vi "publish status.vi"(8 "error in (no error)":errorcluster, 11 "Channel in":refnum<class "Channel.lvclass">) -> (0 "error out":errorcluster, 3 "Channel out":refnum<class "Channel.lvclass">)   [LabVIEW 2018, in "Channel.lvclass"]
uses:
  Channel.lvclass
  Channel.lvclass/Channel.ctl
  State Machine/CCS_State Machine.lvclass/CCS_State Machine.ctl
  State Machine/CCS_State Machine.lvclass
  Simulated_CCD_Camera/Simulated Camera.lvclass
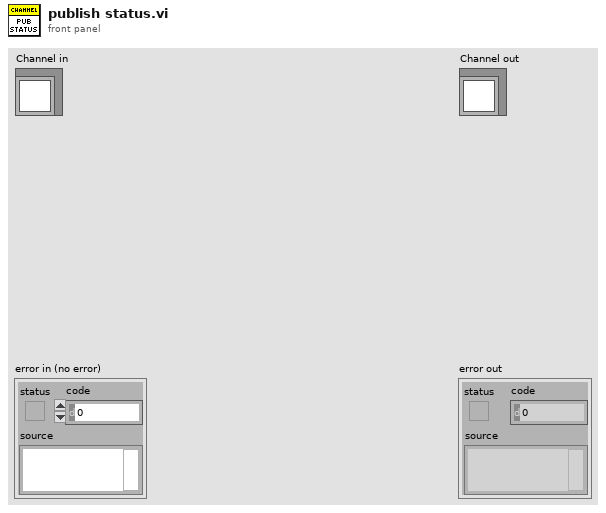
[diagram p1: front panel]
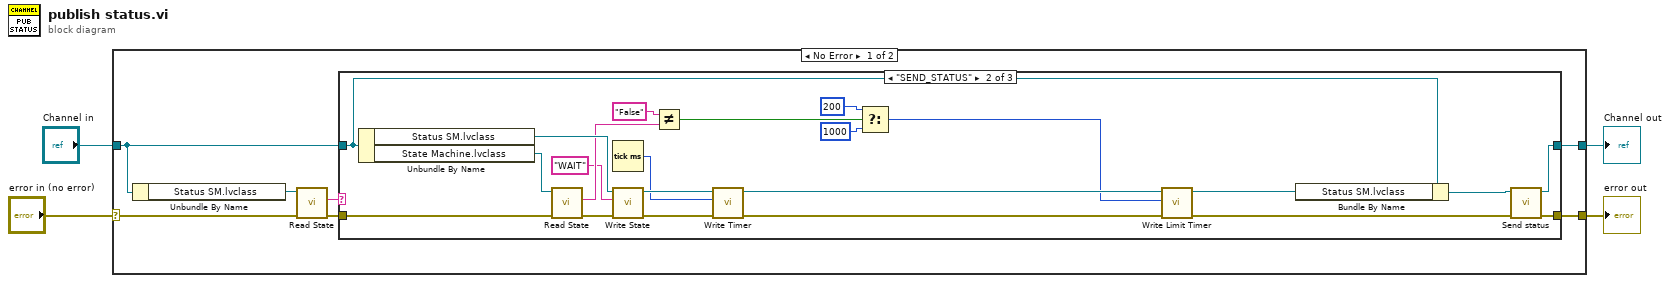
[diagram p0: block diagram]
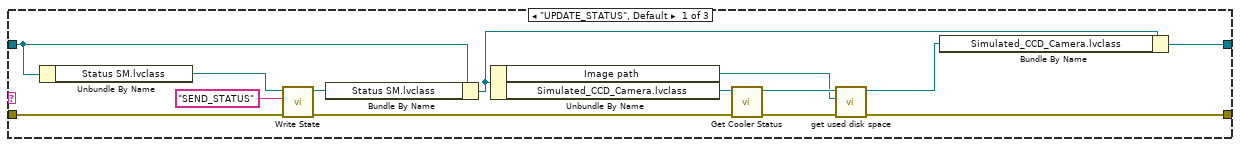
[diagram p2: hidden frame]
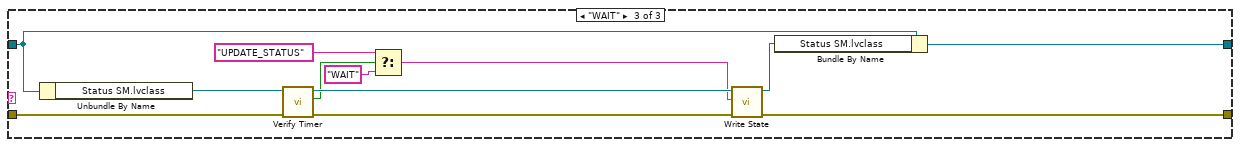
[diagram p3: hidden frame]
diagram:
  n1 = case shown="No Error" "error in (no error)" {
    selector: "error in (no error)" -> [w10 w61]
    tunnel: [w5 w61] -> w3
    tunnel: [w7 w60] -> w1
    tunnel: "Channel in" -> [w6 w60]
    frame No Error {
      n2 = Unbundle By Name(w6) -> ("Status SM.lvclass"=w11:refnum<class "CCS_State Machine.lvclass">)
      n3 = call-dynamic "Read State.vi"("error in (no error)"=w10, "State Machine in"=w11) -> ("error out"=w8:errorcluster, "State"=w9:string)  [unwired: 7 in, 1 out]
      n4 = case shown="\"SEND_STATUS\"" w9 {
        tunnel: w6 -> [w20 w31 w58]
        tunnel: w8 -> [w21 w32 w59]
        tunnel: [w13 w27 w52] -> w5
        tunnel: [w19 w26 w56] -> w7
        frame "UPDATE_STATUS", Default {
          n5 = Unbundle By Name(w20) -> ("Status SM.lvclass"=w23:refnum<class "CCS_State Machine.lvclass">)
          n6 = call-dynamic "Write State.vi"("error in (no error)"=w21, "State"="SEND_STATUS", "State Machine in"=w23) -> ("error out"=w17:errorcluster, "State Machine out"=w24:refnum<class "CCS_State Machine.lvclass">)  [unwired: 7 in]
          n7 = Bundle By Name(cluster=w20, "Status SM.lvclass"=w24) -> (w25:refnum<class "Channel.lvclass">)
          n8 = Unbundle By Name(w25) -> ("Image path"=w12:path, "Simulated_CCD_Camera.lvclass"=w18:refnum<class "Simulated Camera.lvclass">)
          n9 = call-dynamic "Get Cooler Status.vi"("error in (no error)"=w17, "CCDCamera in"=w18) -> ("error out"=w16:errorcluster, "CCDCamera out"=w15:refnum<class "Simulated Camera.lvclass">)  [unwired: 8 in]
          n10 = call "get used disk space.vi"("error in (no error)"=w16, "image path"=w12, "Simulated Camera in"=w15) -> ("error out"=w13:errorcluster, "Simulated Camera out"=w14:refnum<class "Simulated Camera.lvclass">)  [unwired: 7 in]
          n11 = Bundle By Name(cluster=w25, "Simulated_CCD_Camera.lvclass"=w14) -> (w19:refnum<class "Channel.lvclass">)
        }
        frame "SEND_STATUS" {
          n12 = Unbundle By Name(w31) -> ("Status SM.lvclass"=w40:refnum<class "CCS_State Machine.lvclass">, "State Machine.lvclass"=w41:refnum<class "CCS_State Machine.lvclass">)
          n13 = call-dynamic "Read State.vi"("error in (no error)"=w32, "State Machine in"=w41) -> ("error out"=w39:errorcluster, "State"=w38:string)  [unwired: 7 in, 1 out]
          n14 = Tick Count (ms)() -> (millisecond timer value=w45:u32)
          n15 = call-dynamic "Write State.vi"("error in (no error)"=w39, "State"="WAIT", "State Machine in"=w40) -> ("error out"=w46:errorcluster, "State Machine out"=w47:refnum<class "CCS_State Machine.lvclass">)  [unwired: 7 in]
          n16 = Not Equal?(x="False" ("State"), y=w38) -> (x != y?=w30:bool)
          n17 = call "Write Timer.vi"("error in (no error)"=w46, "Timer"=w45, "State Machine in"=w47) -> ("error out"=w42:errorcluster, "State Machine out"=w44:refnum<class "CCS_State Machine.lvclass">)  [unwired: 7 in]
          n18 = Select(t=200, s=w30, f=1000) -> (s? t:f=w37:i32)
          n19 = call "Write Limit Timer.vi"("error in (no error)"=w42, "Limit Timer"=w37, "State Machine in"=w44) -> ("error out"=w28:errorcluster, "State Machine out"=w43:refnum<class "CCS_State Machine.lvclass">)  [unwired: 7 in]
          n20 = Bundle By Name(cluster=w31, "Status SM.lvclass"=w43) -> (w29:refnum<class "Channel.lvclass">)
          n21 = call "Send status.vi"("error in (no error)"=w28, "Channel in"=w29) -> ("error out"=w27:errorcluster, "Channel out"=w26:refnum<class "Channel.lvclass">)  [unwired: 8 in]
        }
        frame "WAIT" {
          n22 = Unbundle By Name(w58) -> ("Status SM.lvclass"=w57:refnum<class "CCS_State Machine.lvclass">)
          n23 = call "Verify Timer.vi"("error in (no error)"=w59, "State Machine in"=w57) -> ("error out"=w55:errorcluster, "time out"=w48:bool, "State Machine out"=w54:refnum<class "CCS_State Machine.lvclass">)  [unwired: 7 in]
          n24 = Select(t="UPDATE_STATUS", s=w48, f="WAIT") -> (s? t:f=w51:string)
          n25 = call-dynamic "Write State.vi"("error in (no error)"=w55, "State"=w51, "State Machine in"=w54) -> ("error out"=w52:errorcluster, "State Machine out"=w53:refnum<class "CCS_State Machine.lvclass">)  [unwired: 7 in]
          n26 = Bundle By Name(cluster=w58, "Status SM.lvclass"=w53) -> (w56:refnum<class "Channel.lvclass">)
        }
      }
    }
    frame Error {
    }
  }
  "error out" <- w3
  "Channel out" <- w1
